vi "Image_Snap_Enqueue.vi"(0 "input cluster":T2={"system"={"info"={"menuSelect"=0, "version"=0, "serial"="Test Sample", "captureActive"=TRUE, "captureBegin"=TRUE, "emptyAndRefill"=TRUE}, "userInfo"={"operatorName"="", "date"=timestamp(2713993200 s since 1904-01-01)}, "camera"={"exposureTime"=0, "aperture"=enum."Item 0", "framerate"=0, "framerateMax"=500, "legacyAttributes"=TRUE}}, "connections"={"arduino"={"connection"="First test samples", "status"=TRUE, "openState"=FALSE, "emptyStart"=0}, "pump"={"connection"="MRJ", "status"=TRUE, "command"="", "dispenseSpeed"=100, "flushSize"=100}, "camera"={"cam1"={"connection"="", "status"=FALSE}, "cam2"={"connection"="", "status"=FALSE}}}, "queue"={"process"={"cam1"=refnum, "cam2"=refnum, "queueSize"=0}, "save"={"cam1"=refnum, "cam2"=refnum, "queueSize"=0}, "overloadThreshold"=0}, "imageProcess"={"cam1"={"preAllocation"={"image"="Station", "originalDisplay"="Station", "originalRgb"="Station", "binary"="Station", "save"="Station", "calibrationFull"="remote image 0000000015E6FBB4", "calibrationDetect"="remote image 0000000015E6F134"}, "calibration"={"pathFull"=path "C:/Users/au540322/Desktop/IHS_Project/calibration/Test Calibration/Test Calibration_7/1Test Calibration_7_2019_06_07-23-38-32-452.PNG", "pathDetect"=path "C:/Users/au540322/Desktop/IHS_Project/calibration/Test Calibration/Test Calibration_7/2Test Calibration_7_2019_06_07-23-38-32-415.PNG", "ROI"={"Left"=0, "Top"=0, "Right"=0, "Bottom"=0, "Rotation"=0.0}}}, "cam2"={"preAllocation"={"image"=refnum, "originalDisplay"=refnum, "originalRgb"=refnum, "binary"=refnum, "save"=refnum, "calibrationFull"=refnum, "calibrationDetect"=refnum}, "calibration"={"pathFull"=path "C:/Users/au540322/Desktop/IHS_Project/images/Debris/Debris_0/Debris_0_2019_06_01-23-32-49-686.PNG", "pathDetect"=path "C:/Users/au540322/Desktop/IHS_Project/images/Debris/Debris_0/Debris_0_2019_06_01-23-32-49-686.PNG", "ROI"={"Left"=0, "Top"=0, "Right"=0, "Bottom"=0, "Rotation"=0.0}}}, "process"={"planeExtract"=refnum, "planeSubtract"=refnum, "cropMask"=refnum}, "detection"={"sampleTimeout"=500, "sizeThreshold"=500, "detectionRegionPct"=0.0}}, "sampleData"={"sampleId"="", "projectId"="", "voucherID"="", "speciesName"="", "collectionDate"=timestamp(2713993200 s since 1904-01-01), "sampleStation"="", "location"="", "lat"=0.0, "lon"=0.0, "determiner"="", "sex"="", "otherNotes"=""}, "Session In"=""} {"sampleData"."collectionDate" format="%<%Y-%m-%d>T"; "imageProcess"."detection"."sizeThreshold" min=1; "imageProcess"."cam2"."calibration"."ROI"."Rotation" format="%.2f"; "imageProcess"."cam2"."calibration"."ROI"."Left" scale=0.0..1024.0; "imageProcess"."cam2"."calibration"."ROI"."Right" scale=0.0..1024.0; "imageProcess"."cam1"."calibration"."ROI"."Rotation" format="%.2f"; "imageProcess"."cam1"."calibration"."ROI"."Left" scale=0.0..1024.0; "imageProcess"."cam1"."calibration"."ROI"."Right" scale=0.0..1024.0; "queue"."overloadThreshold" min=1; "queue"."save"."queueSize" min=1; "queue"."process"."queueSize" min=1; "connections"."pump"."flushSize" min=1; "connections"."pump"."dispenseSpeed" min=1; "system"."camera"."framerateMax" min=1; "system"."userInfo"."date" format="%<%Y-%m-%dT%H:%M:%S+%z>T"; "system"."info"."version" items=["Standard", "XL"]; "system"."info"."menuSelect" items=["Session Data", "Extended Setup", "Buffer", "Camera", "Dispenser", "Stats", "Connections"]}, 5 "Camera queue":refnum<queue>, 7 "Camera":T1, 9 "Detect Movement":bool, 11 "error in":errorcluster) -> (4 "Image out":T4, 15 "error out":errorcluster)   [LabVIEW 2022 SP3]
doc: "Takes picture from single camera and converts to array output."
uses:
  <vilib>/vision/Image Controls.llb/IMAQ Image.ctl
  controls/Data.ctl
  <vilib>/userdefined/High Color/IMAQdx.ctl
  Camera_ID.ctl
  <vilib>/vision/driver/NI_Vision_Acquisition_Software.lvlib
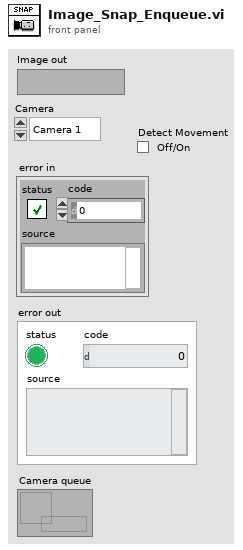
[diagram p1: front panel]
types:
  T1 = typedef "Camera_ID.ctl" = enum16{"Camera 1", "Camera 2"}
  T2 = typedef "Data.ctl" = cluster{"system":cluster{"info":cluster{"menuSelect":u16, "version":u16, "serial":string, "captureActive":bool, "captureBegin":bool, "emptyAndRefill":bool}, "userInfo":cluster{"operatorName":string, "date":timestamp}, "camera":cluster{"exposureTime":i32, "aperture":enum32{"Item 0", "Item 1", "Item 2", "Item 3"}, "framerate":i32, "framerateMax":i32, "legacyAttributes":bool}}, "connections":cluster{"arduino":cluster{"connection":refnum<visa-resource-name>, "status":bool, "openState":bool, "emptyStart":u32}, "pump":cluster{"connection":refnum<visa-resource-name>, "status":bool, "command":string, "dispenseSpeed":i32, "flushSize":i32}, "camera":cluster{"cam1":cluster{"connection":T3, "status":bool}, "cam2":cluster{"connection":T3, "status":bool}}}, "queue":cluster{"process":cluster{"cam1":refnum<queue>, "cam2":refnum<queue>, "queueSize":i32}, "save":cluster{"cam1":refnum<queue>, "cam2":refnum<queue>, "queueSize":i32}, "overloadThreshold":i32}, "imageProcess":cluster{"cam1":cluster{"preAllocation":cluster{"image":T4, "originalDisplay":T4, "originalRgb":T4, "binary":T4, "save":T4, "calibrationFull":T4, "calibrationDetect":T4}, "calibration":cluster{"pathFull":path, "pathDetect":path, "ROI":T5}}, "cam2":cluster{"preAllocation":cluster{"image":T4, "originalDisplay":T4, "originalRgb":T4, "binary":T4, "save":T4, "calibrationFull":T4, "calibrationDetect":T4}, "calibration":cluster{"pathFull":path, "pathDetect":path, "ROI":T5}}, "process":cluster{"planeExtract":T4, "planeSubtract":T4, "cropMask":T4}, "detection":cluster{"sampleTimeout":i32, "sizeThreshold":i32, "detectionRegionPct":dbl}}, "sampleData":cluster{"sampleId":string, "projectId":string, "voucherID":string, "speciesName":string, "collectionDate":timestamp, "sampleStation":string, "location":string, "lat":dbl, "lon":dbl, "determiner":string, "sex":string, "otherNotes":string}, "Session In":T3}
  T3 = typedef "IMAQdx.ctl" = refnum<k21>
  T4 = typedef "IMAQ Image.ctl" = refnum<image>
  T5 = typedef "IMAQ Rectangle" = cluster{"Left":i32, "Top":i32, "Right":i32, "Bottom":i32, "Rotation":dbl}
  T6 = cluster{"Image Pixels (U32)":u32[][], "Detect Movement":bool}
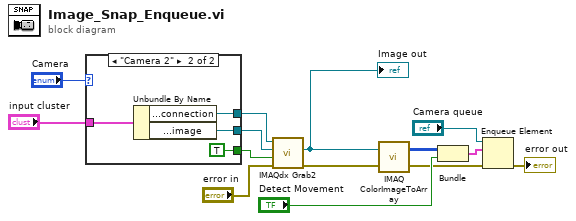
[diagram p0: block diagram]
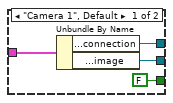
[diagram p2: hidden frame]
diagram:
  n1 = case shown="\"Camera 2\"" "Camera" {
    tunnel: "input cluster" -> [w16 w22]
    tunnel: [w18 w21] -> w8
    tunnel: [w17 w20] -> w13
    tunnel: [FALSE ("Wait for Next Buffer? (Yes)") TRUE ("Wait for Next Buffer? (Yes)")] -> w9
    frame "Camera 1", Default {
      n2 = Unbundle By Name(w16) -> ("connections.camera.cam1.connection"=w18:T3, "imageProcess.cam1.preAllocation.image"=w17:T4)
    }
    frame "Camera 2" {
      n3 = Unbundle By Name(w22) -> ("connections.camera.cam2.connection"=w21:T3, "imageProcess.cam2.preAllocation.image"=w20:T4)
    }
  }
  n4 = call <vilib>:"IMAQdx Grab2.vi"("error in"="error in", "Wait for Next Buffer? (Yes)"=w9, "Image In"=w13, "Session In"=w8) -> ("error out"=w3:errorcluster, "Image Out"=w4:T4)  [unwired: 4 in, 2 out]
  "Image out" <- w4
  n5 = call "IMAQ ColorImageToArray"("Image"=w4, "error in (no error)"=w3) -> ("Image Pixels (U32)"=w2:u32[][], "error out"=w5:errorcluster)  [unwired: 2 in, 1 out]
  n6 = Bundle("Image Pixels (U32)"=w2, "Detect Movement"="Detect Movement") -> (w6:T6)  [unwired: 1 in]
  n7 = Enqueue Element(queue="Camera queue", element=w6, error in (no error)=w5) -> (error out=→"error out":errorcluster)  [unwired: 1 in, 2 out]
